vi "Producer Consumer Events Labview VS Arduino.vi"() -> ()   [LabVIEW 2018]
doc: "Use this template to build a producer/consumer design pattern with events to produce queue items. Use this design pattern instead of the User Interface Event Handler pattern for user interfaces when you want to execute code asynchronously in response to an event without slowing the user interface responsiveness."
panel:
  out "DIGITAL 1":bool
  out "DIGITAL 0":bool
  out "Waveform Chart":T1(graph)
  out "error out":errorcluster
  in  "pin2 state":bool
  in  "pin4 state":bool
  in  "ANOLOG OUTPUT [ PWM]":u16(knob) scale=0.0..255.0
  out "data (can be any type)":string
  in  "Serial USB com ARUINO port":refnum<visa-resource-name>="COM3"
  in  "send configuration":bool
  in  "enable DIO":bool
  in  "Digital (pin2) conf":enum32{"Item 0", "Item 1"}(radio)
  in  "Digital (pin4) conf":enum32{"Item 0", "Item 1"}(radio)
  in  "Ts (Sampling Rate)":u16(ring) items=["1000 sec"=0, "100 msec"=8, "10 msec"=4, "1 msec"=2, "500 usec"=1]
  in  "A5":bool
  in  "A4":bool
  in  "A3":bool
  in  "A2":bool
  in  "A1":bool
  in  "A0":bool
  in  "stop":bool
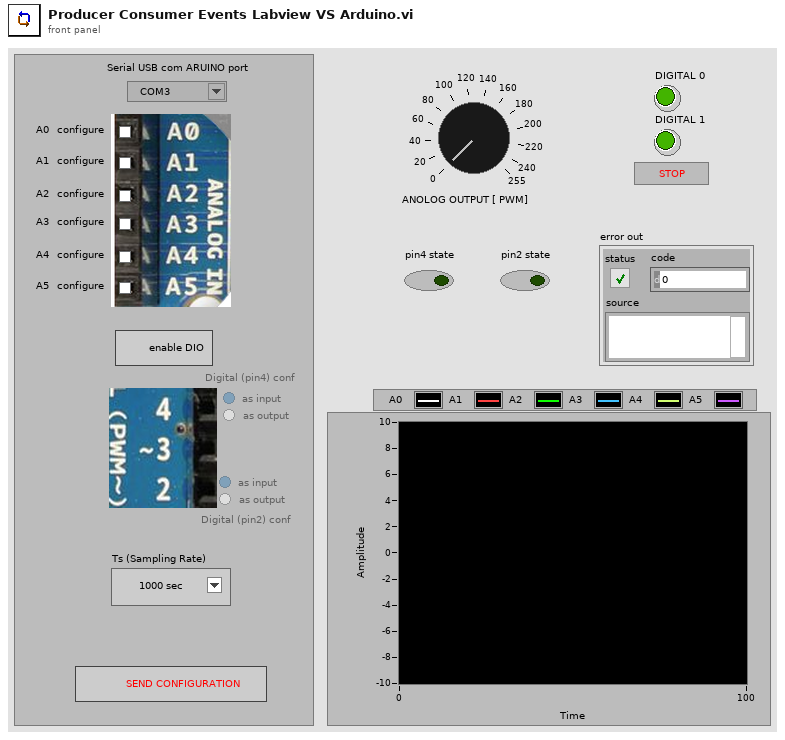
[diagram p1: front panel]
types:
  T1 = cluster{"[0]":dbl, "[1]":dbl, "[2]":dbl, "[3]":dbl, "[4]":dbl, "[5]":dbl, "[6]":dbl, "[7]":dbl, "[8]":dbl}
  T2 = enum8{"Enabled", "Disabled", "Disabled and Grayed Out"}
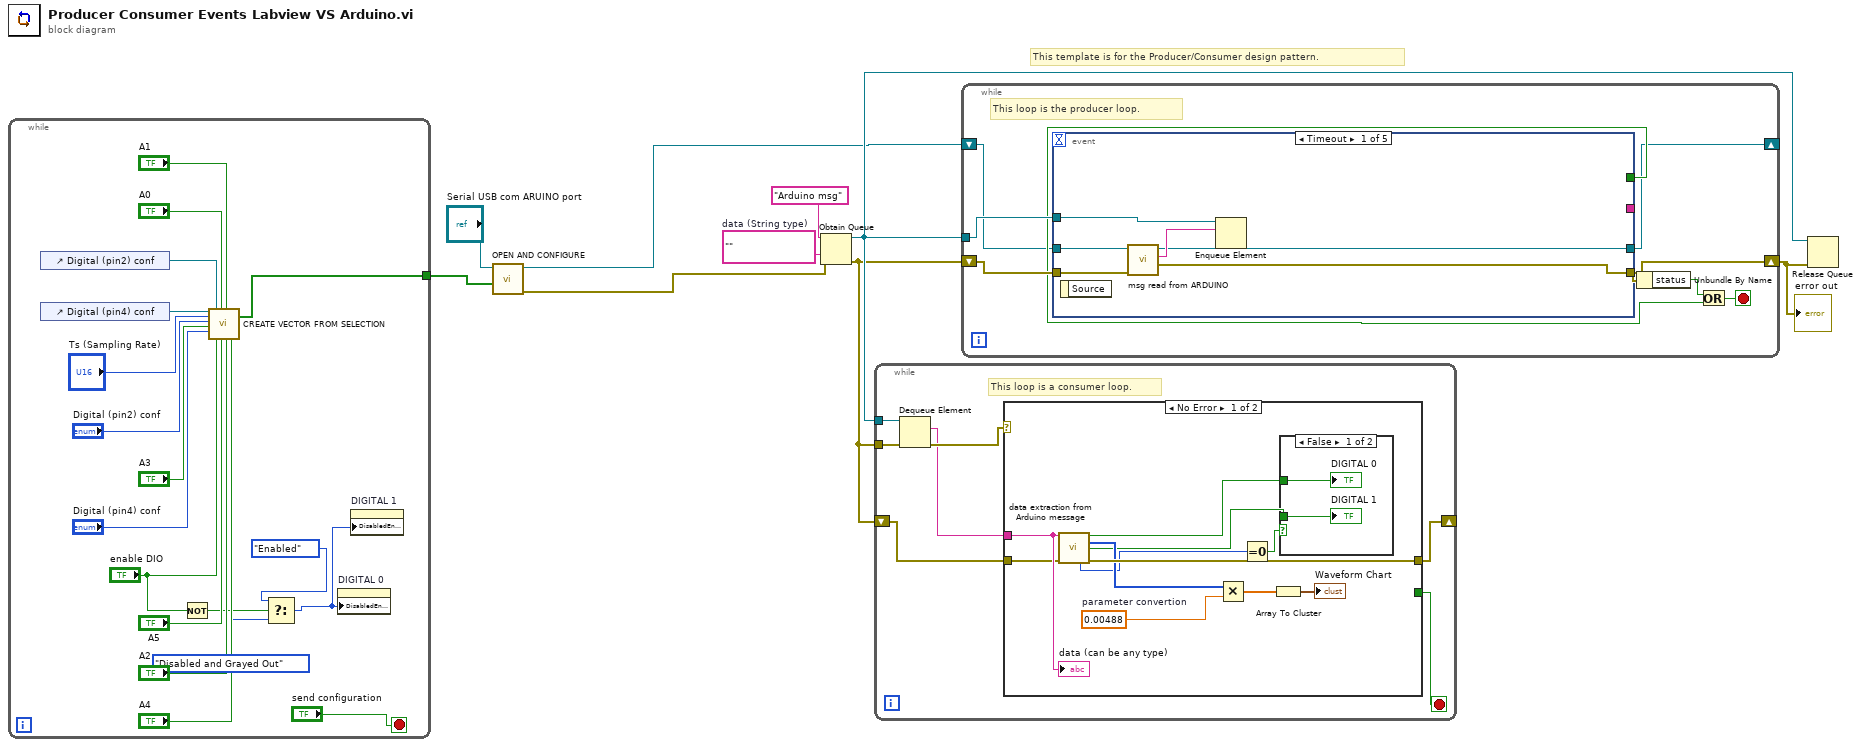
[diagram p0: block diagram]
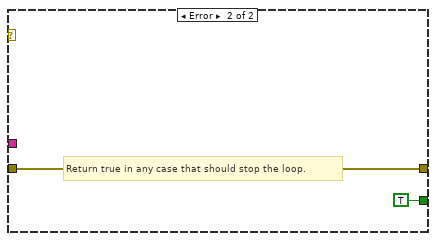
[diagram p3: hidden frame]
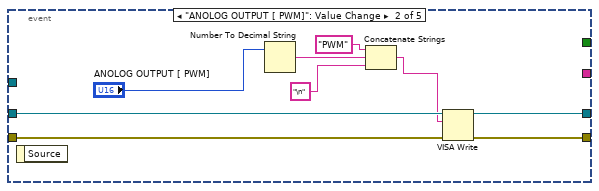
[diagram p4: hidden frame]
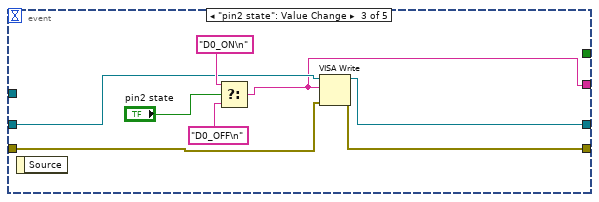
[diagram p5: hidden frame]
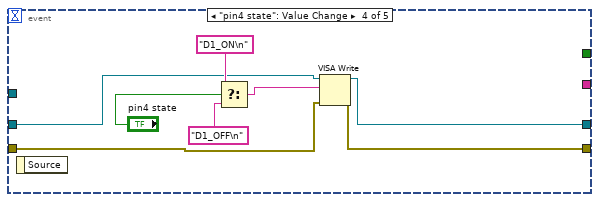
[diagram p6: hidden frame]
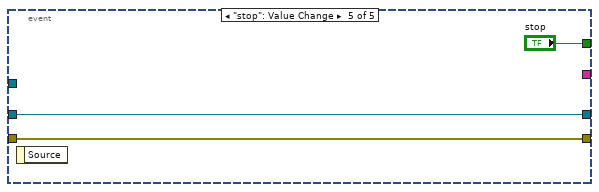
[diagram p7: hidden frame]
diagram:
  w8 = ""  # data (String type)
  # "This template is for the Producer/Consumer design pattern."
  n1 = while {
    tunnel: [w19] -> w6
    stop <- "send configuration" stop-if-true
    n2 = control-ref of="Digital (pin2) conf"() -> (w15:refnum<vi>)
    n3 = control-ref of="Digital (pin4) conf"() -> (w16:refnum<vi>)
    n4 = Not(x="enable DIO") -> (.not. x?=w11:bool)
    n5 = call "CREATE VECTOR FROM SELECTION.vi"("RadioButtonsControl in"=w16, "Ts (Sampling Rate)"="Ts (Sampling Rate)", "Digital (pin2) conf"="Digital (pin2) conf", "A3"="A3", "Digital (pin4) conf"="Digital (pin4) conf", "RadioBtnsControl Refnum in"=w15, "enable DIO"="enable DIO", "A0"="A0", "A5"="A5", "A1"="A1", "A2"="A2", "A4"="A4") -> ("Array"=w19:bool[])  [unwired: 7 in]
    n6 = Select(t=T2."Enabled" ("Disabled"), s=w11, f=T2."Disabled and Grayed Out" ("Disabled")) -> (s? t:f=w10:T2)
    n7 = property on="DIGITAL 0" class="Bool (strict)"("DisabledEnum"=w10) -> ()  [unwired: 2 in, 2 out]
    n8 = property on="DIGITAL 1" class="Bool (strict)"("DisabledEnum"=w10) -> ()  [unwired: 2 in, 2 out]
  }
  n9 = call "OPEN AND CONFIGURE.vi"("array configuration"=w6, "VISA resource name"="Serial USB com ARUINO port") -> ("error out SERIAL OPEN"=w5:errorcluster, "VISA resource name out"=w3:refnum<visa-resource-name>)  [unwired: 7 in, 1 out]
  n10 = Obtain Queue(name (unnamed)="Arduino msg", element data type=w8, error in (no error)=w5) -> (queue out=w7:refnum<queue>, error out=w1:errorcluster)  [unwired: 2 in, 1 out]
  n11 = while {
    tunnel: w7 -> [w34]
    shift-right: [w29] -> _
    shift-left: w1 -> [w30]
    tunnel: w1 -> [w28]
    stop <- w31 stop-if-true
    # "This loop is a consumer loop."
    n12 = Dequeue Element(queue=w34, error in (no error)=w28) -> (element=w32:string, error out=w33:errorcluster)  [unwired: 1 in, 2 out]
    n13 = case shown="No Error" w33 {
      tunnel: w32 -> [w45 _]
      tunnel: [_ TRUE] -> w31
      tunnel: w30 -> [w44 w48]
      tunnel: [w43 w48] -> w29
      frame No Error {
        w41 = 0.00488  # parameter convertion
        n14 = call "data extraction from Arduino message.vi"("data (can be any type)"=w45, "error IO"=w44) -> ("DIn 0"=w38:bool, "Analog channel reading"=w42:u32[], "DIn 1"=w37:bool, "size digital array"=w40:i32, "error out"=w43:errorcluster)  [unwired: 7 in, 2 out]
        n15 = Multiply(x=w42, y=w41) -> (x*y=w36:dbl[])
        n16 = Equal To 0?(x=w40) -> (x = 0?=w39:bool)
        n17 = Array To Cluster(array=w36) -> (cluster=→"Waveform Chart":T1)
        n18 = case shown="False" w39 {
          tunnel: w38 -> [w47 _]
          tunnel: w37 -> [w46 _]
          frame False {
            "DIGITAL 1" <- w46
            "DIGITAL 0" <- w47
          }
          frame True {
          }
        }
        "data (can be any type)" <- w45
      }
      frame Error {
        # "Return true in any case that should stop the loop."
      }
    }
  }
  n19 = while {
    shift-right: [w53] -> w9
    shift-left: w1 -> [w56]
    tunnel: w7 -> [w57]
    shift-right: [w50] -> _
    shift-left: w3 -> [w51]
    stop <- w54 stop-if-true
    # "This loop is the producer loop."
    n20 = event shown="[0] Timeout" {
      selector: _ -> [_ _ _ _ _]
      dyn-events: _ -> [_ _ _ _ _]
      timeout: _ -> [_ _ _ _ _]
      tunnel: w57 -> [w60 _ _ _ _]
      tunnel: w56 -> [w62 w71 w74 w83 w90]
      tunnel: [w61 w70 w75 w84 w90] -> w53
      tunnel: [_ _ _ _ "stop"] -> w55
      tunnel: w51 -> [w63 w72 w77 w86 w89]
      tunnel: [w58 w69 w76 w85 w89] -> w50
      tunnel: [_ _ w73 _ _] -> _
      event Timeout {
        n21 = event-data() -> ()  [unwired: 1 in, 1 out]
        n22 = call "msg read from ARDUINO.vi"("error in (read msg)"=w62, "VISA Refnum in"=w63) -> ("error out (read msg)"=w61:errorcluster, "msg answer"=w59:string, "VISA Refnum out"=w58:refnum<visa-resource-name>)  [unwired: 7 in]
        n23 = Enqueue Element(queue=w60, element=w59) -> ()  [unwired: 2 in, 3 out]
      }
      event "ANOLOG OUTPUT [ PWM]": Value Change {
        n24 = event-data() -> ()  [unwired: 1 in, 1 out]
        n25 = Number To Decimal String(number="ANOLOG OUTPUT [ PWM]") -> (decimal integer string=w67:string)  [unwired: 1 in]
        n26 = Concatenate Strings("PWM" ("string"), w67, "\n" ("element")) -> (w64:string)
        n27 = VISA Write(VISA resource name=w72, write buffer=w64, error in (no error)=w71) -> (VISA resource name out=w69:refnum<visa-resource-name>, error out=w70:errorcluster)  [unwired: 1 out]
      }
      event "pin2 state": Value Change {
        n28 = event-data() -> ()  [unwired: 1 in, 1 out]
        n29 = Select(t="D0_ON\n", s="pin2 state", f="D0_OFF\n") -> (s? t:f=w73:string)
        n30 = VISA Write(VISA resource name=w77, write buffer=w73, error in (no error)=w74) -> (VISA resource name out=w76:refnum<visa-resource-name>, error out=w75:errorcluster)  [unwired: 1 out]
      }
      event "pin4 state": Value Change {
        n31 = event-data() -> ()  [unwired: 1 in, 1 out]
        n32 = Select(t="D1_ON\n", s="pin4 state", f="D1_OFF\n") -> (s? t:f=w81:string)
        n33 = VISA Write(VISA resource name=w86, write buffer=w81, error in (no error)=w83) -> (VISA resource name out=w85:refnum<visa-resource-name>, error out=w84:errorcluster)  [unwired: 1 out]
      }
      event "stop": Value Change {
        n34 = event-data() -> ()  [unwired: 1 in, 1 out]
      }
    }
    n35 = Unbundle By Name(w53) -> ("status"=w52:bool)
    n36 = Or(x=w52, y=w55) -> (x .or. y?=w54:bool)
  }
  "error out" <- w9
  n37 = Release Queue(queue=w7, error in (no error)=w9) -> ()  [unwired: 1 in, 3 out]
